vi "mqttCmdBuildPayload.vi"(0 "_mqtt in":refnum<class "mqttCmdPublish.lvclass">, 11 "error in (no error)":errorcluster) -> (4 "_mqtt out":refnum<class "mqttCmdPublish.lvclass">, 8 "payload":u8[](array[numeric]) format="%x", 15 "error out":errorcluster)   [LabVIEW 2019, in "mqttCmdPublish.lvclass"]
uses:
  mqttCmdPublish.lvclass
  mqttCmdPublish.lvclass/mqttCmdPublish.ctl
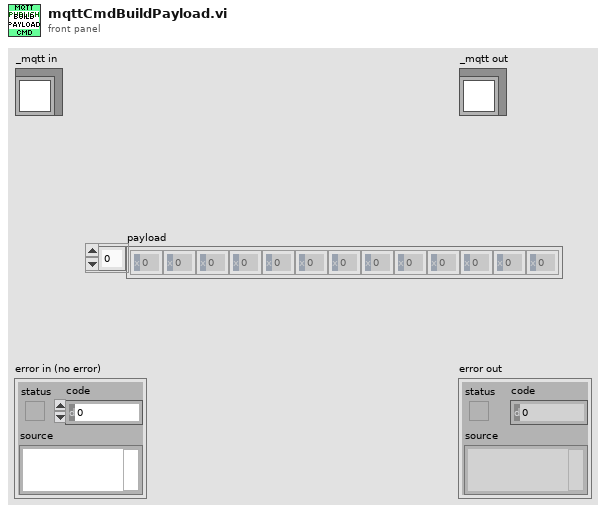
[diagram p1: front panel]
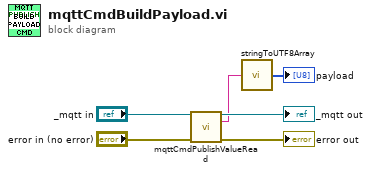
[diagram p0: block diagram]
diagram:
  n1 = call "mqttCmdPublishValueRead.vi"("mqttPublish in"="_mqtt in", "error in (no error)"="error in (no error)") -> ("mqttPublish out"=→"_mqtt out":refnum<class "mqttCmdPublish.lvclass">, "value"=w2:string, "error out"=→"error out":errorcluster)  [unwired: 11 in]
  n2 = call "stringToUTF8Array.vi"("string"=w2) -> ("UTF8[]"=→"payload":u8[])  [unwired: 14 in]
